vi "Pre Launch Init.vi"(11 "启动器 in":refnum<class "启动器.lvclass"> caption="操作者输入") -> (0 "error out":errorcluster caption="错误输出", 3 "启动器 out":refnum<class "启动器.lvclass"> caption="操作者输出")   [LabVIEW 2017, in "启动器.lvlib" / "启动器.lvclass"]
doc: "(<B>Filename</B>: Actor Framework.lvlib:Actor.lvclass:Pre Launch Init.vi)\n\nDefines behavior that occurs after the Launch Nested Actor method is invoked but before the actor's Actor Core method begins running.\n\nBy default, this method does nothing. A descendant class may override it to define behavior."
uses:
  <vilib>/ActorFramework/Actor/Actor.lvclass
  <vilib>/Utility/config.llb/NI_LVConfig.lvlib
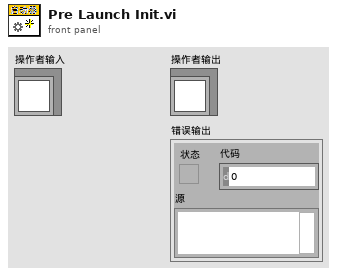
[diagram p1: front panel]
types:
  T1 = typedef "NI_LVConfig.lvlib/Config Data RefNum.ctl" = refnum<k1>
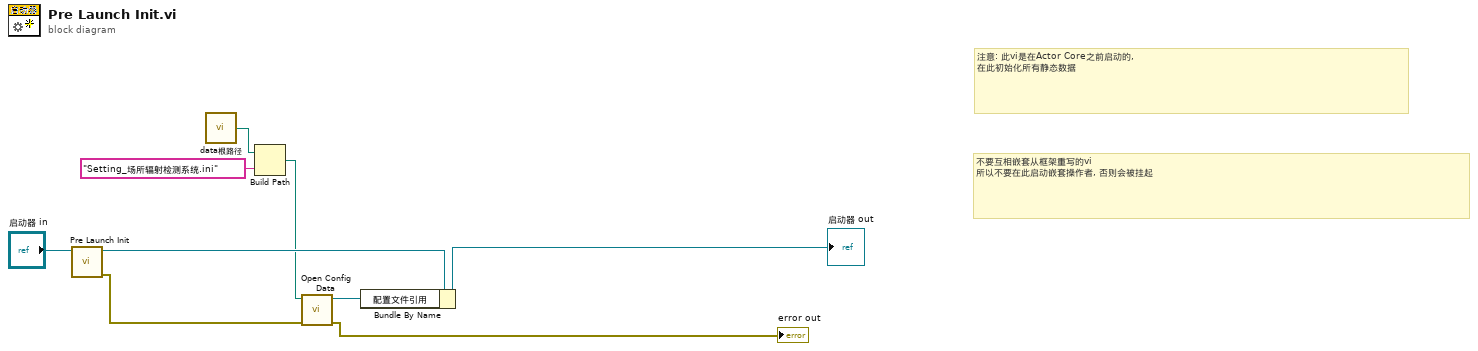
[diagram p0: block diagram]
diagram:
  # "不要互相嵌套从框架重写的vi\n所以不要在此启动嵌套操作者, 否则会被挂起"
  # "注意: 此vi是在Actor Core之前启动的, \n在此初始化所有静态数据"
  n1 = call-parent "Pre Launch Init.vi"("Actor in"="启动器 in") -> ("error out"=w2:errorcluster, "Actor out"=w9:refnum<class "启动器.lvclass">)  [unwired: 9 in]
  n2 = call "data根路径.vi"() -> ("data文件夹"=w7:path)
  n3 = Build Path(base path=w7, name or relative path="Setting_场所辐射检测系统.ini" ("名称或相对路径")) -> (appended path=w5:path)
  n4 = call <vilib>:"Open Config Data.vi"("error in (no error)"=w2, "configuration file path"=w5) -> ("error out"=→"error out":errorcluster, "refnum"=w3:T1)  [unwired: 7 in, 1 out]
  n5 = Bundle By Name(cluster=w9, "配置文件引用"=w3) -> (→"启动器 out":refnum<class "启动器.lvclass">)
